vi "Publish.vi"(8 "error in (no error)":errorcluster, 10 "PublishRequest":refnum<class "PublishRequest.lvclass">, 11 "Mediator in":refnum<class "Mediator.lvclass">) -> (0 "error out":errorcluster, 3 "Mediator out":refnum<class "Mediator.lvclass">)   [LabVIEW 2018, in "MVA Framework.lvlib" / "Mediator.lvlib" / "Mediator.lvclass"]
doc: "发布"
uses:
  Mediator.lvclass
  TopicLookupTable/TopicLookupTable.lvclass
  Topic Messages/Notify Subscribers Msg/Notify Subscribers Msg.lvclass
  IMediator/PublishRequest/PublishRequest.lvclass
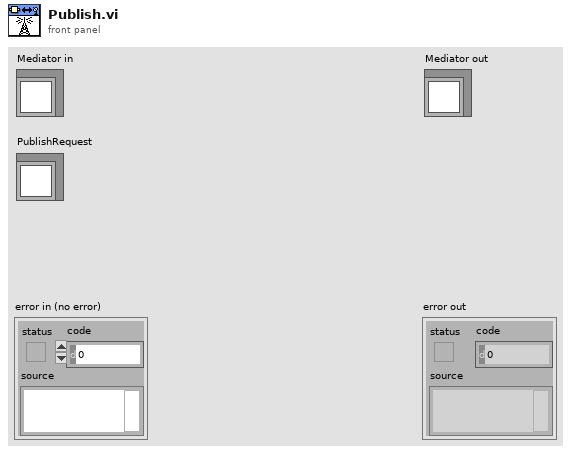
[diagram p1: front panel]
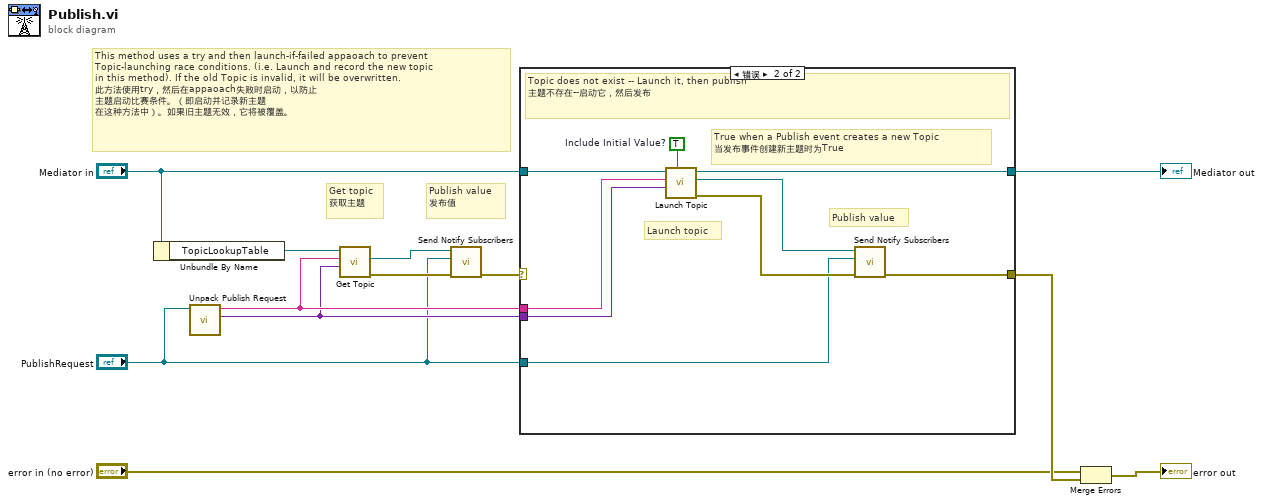
[diagram p0: block diagram]
diagram:
  # "Get topic\n获取主题"
  # "This method uses a try and then launch-if-failed appaoach to prevent\nTopic-launching race conditions. (i.e. Launch and record the new topic\nin this method). If the old Topic is invalid, it will be overwritten.\n此方法使用try，然后在appaoach失败时启动，以防止\n主题启动比赛条件。（即启动并记录新主题\n在这种方法中）。如果旧主题无效，它将被覆盖。"
  # "Publish value\n发布值"
  n1 = Unbundle By Name("Mediator in") -> ("TopicLookupTable"=w2:refnum<data-value>)
  n2 = call "Unpack Publish Request.vi"("PublishRequest In"="PublishRequest") -> ("Value"=w4:variant, "Datum Name"=w5:string)  [unwired: 7 in, 2 out]
  n3 = call "Get Topic.vi"("Topic Type"=w4, "Topic Name"=w5, "TopicLookupTable"=w2) -> ("error out"=w9:errorcluster, "Topic Enqueuer"=w12:refnum<class "Message Enqueuer.lvclass">)  [unwired: 6 in, 1 out]
  n4 = call "Send Notify Subscribers.vi"("error in (no error)"=w9, "PublishRequest"="PublishRequest", "Message Enqueuer"=w12) -> ("error out"=w11:errorcluster)  [unwired: 7 in, 1 out]
  n5 = case shown="错误" w11 {
    selector: w11 -> [w13 _]
    tunnel: "Mediator in" -> [w14 w23]
    tunnel: [w14 w21] -> w8
    tunnel: w5 -> [_ w19]
    tunnel: w4 -> [_ w18]
    tunnel: [w13 w22] -> w10
    tunnel: "PublishRequest" -> [_ w15]
    frame No Error {
      # "Topic exists -- Publish OK\n主题已存在--发布确定"
    }
    frame Error {
      w16 = TRUE  # Include Initial Value?
      # "True when a Publish event creates a new Topic\n当发布事件创建新主题时为True"
      # "Launch topic"
      # "Publish value"
      # "Topic does not exist -- Launch it, then publish\n主题不存在--启动它，然后发布"
      n6 = call-dynamic "Launch Topic.vi"("Include Initial Value? (F)"=w16, "Type"=w18, "Datum Name"=w19, "Mediator in"=w23) -> ("error out"=w17:errorcluster, "New Topic Enqueuer"=w20:refnum<class "Message Enqueuer.lvclass">, "Mediator out"=w21:refnum<class "Mediator.lvclass">)  [unwired: 5 in]
      n7 = call "Send Notify Subscribers.vi"("error in (no error)"=w17, "PublishRequest"=w15, "Message Enqueuer"=w20) -> ("error out"=w22:errorcluster)  [unwired: 7 in, 1 out]
    }
  }
  "Mediator out" <- w8
  n8 = Merge Errors("error in (no error)", w10) -> (→"error out":errorcluster)
